vi "Resistance_SMUResistanceTest.vi"(7 "Published Data Id":T2, 9 "DCPower_Parameters":T1={"Output"=enum."DC Voltage", "Current_range"=0.0, "Current"=0.0, "Voltage_range"=0.0, "Voltage"=0.0, "Aperture_time"=0.0, "Source Delay"=0.0, "Sense"=1008} {"Source Delay" format="%.6p"; "Sense" items=["Local"=1008, "Remote"=1009]; "Aperture_time" format="%.6p"; "Current_range" format="%.6p"; "Current" format="%.6p"; "Voltage_range" format="%.6p"; "Voltage" format="%.6p"}, 10 "Pins":T3[](array[typedef]), 11 "Semiconductor Module Context":T4) -> (0 "error out":errorcluster)   [LabVIEW 2023, in "Resistance.lvlib"]
doc: "Measures the resistance using an SMU channel in order to perform simple Continuity Test"
uses:
  Resistance.lvlib
  <vilib>/NI_TestStand_SemiconductorModule/NI_TestStand_Semiconductor_Module.lvlibp/PinMap/General/SemiconductorModuleContext.ctl
  <vilib>/NI_TestStand_SemiconductorModule/NI_TestStand_Semiconductor_Module.lvlibp/PinMap/TagProvider/TSM_Pin.ctl
  <vilib>/NI_TestStand_SemiconductorModule/NI_TestStand_Semiconductor_Module.lvlibp/PinMap/TagProvider/TSM_PublishedDataId.ctl
  ResourceHandling/TypeDefs/RH_DCPower_Parameters.ctl
  <vilib>/NI_TestStand_SemiconductorModule/NI_TestStand_Semiconductor_Module.lvlibp/PinMap/DC Power/PinsToNIDCPowerSessions.vi
  <vilib>/NI_TestStand_SemiconductorModule/NI_TestStand_Semiconductor_Module.lvlibp/PinMap/General/Publish/PublishDataPerSiteDoubleScalar.vi
  ResourceHandling/ResourceHandling.lvlib
  <vilib>/NI_TestStand_SemiconductorModule/NI_TestStand_Semiconductor_Module.lvlibp
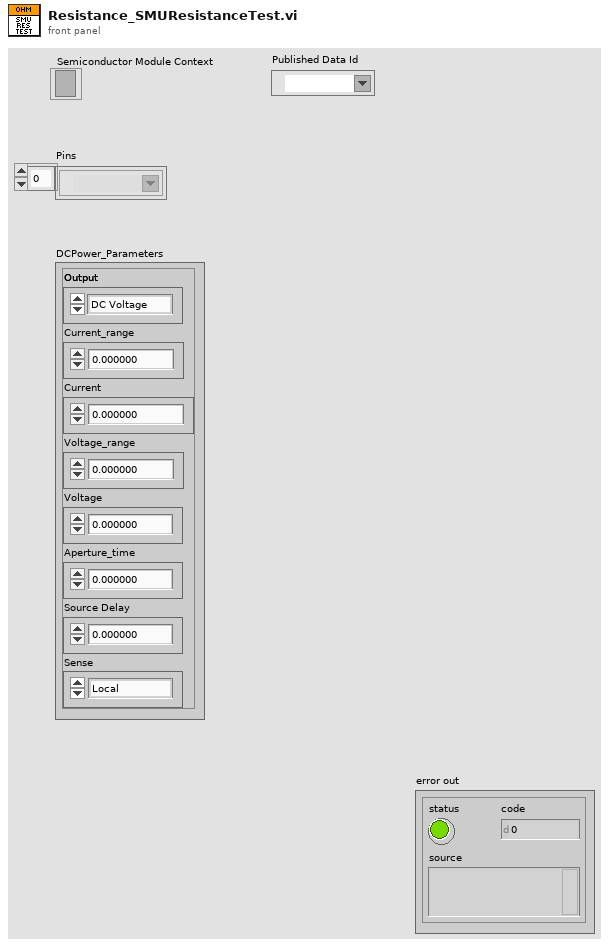
[diagram p1: front panel]
types:
  T1 = typedef "ResourceHandling.lvlib/RH_DCPower_Parameters.ctl" = cluster{"Output":enum16{"DC Voltage", "DC Current"}, "Current_range":dbl, "Current":dbl, "Voltage_range":dbl, "Voltage":dbl, "Aperture_time":dbl, "Source Delay":dbl, "Sense":i32}
  T2 = typedef "NI_TestStand_Semiconductor_Module.lvlibp/TSM_PublishedDataId.ctl" = tag
  T3 = typedef "NI_TestStand_Semiconductor_Module.lvlibp/TSM_Pin.ctl" = tag
  T4 = typedef "NI_TestStand_Semiconductor_Module.lvlibp/SemiconductorModuleContext.ctl" = refnum<k7>
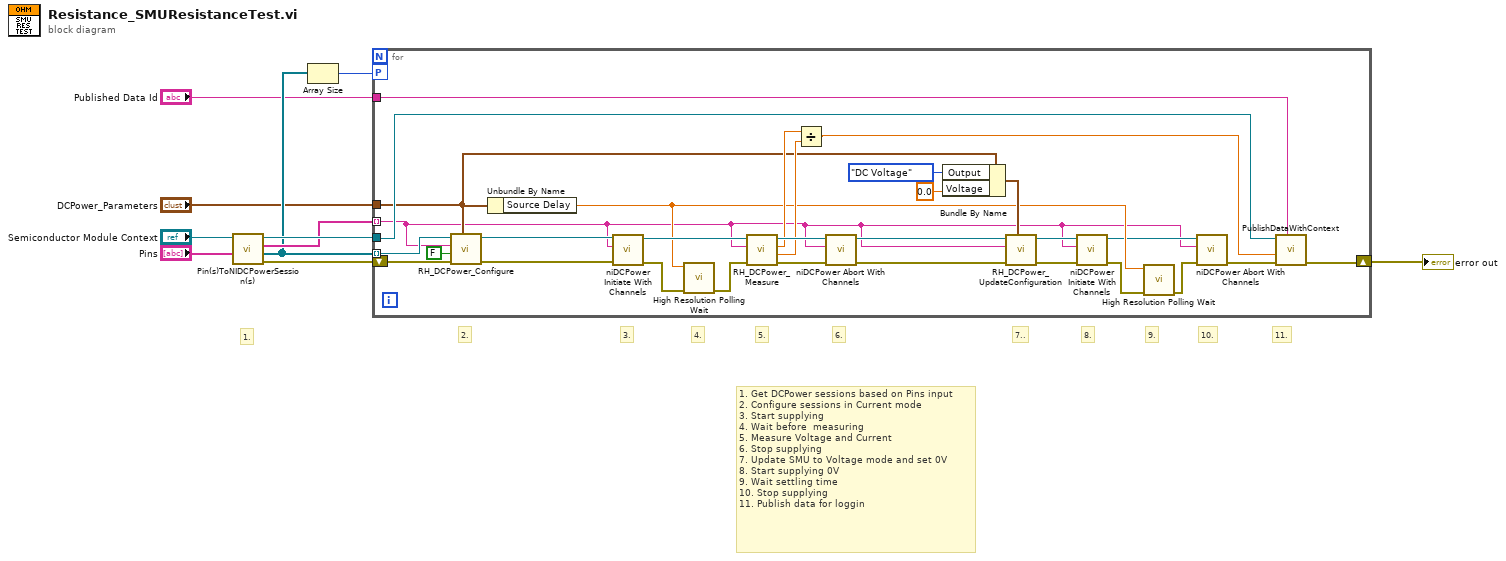
[diagram p0: block diagram]
diagram:
  # "11."
  # "10."
  # "9."
  # "8."
  # "1. Get DCPower sessions based on Pins input\n2. Configure sessions in Current mode\n3. Start supplying\n4. Wait before  measuring\n5. Measure Voltage and Current\n6. Stop supplying\n7. Update SMU to Voltage mode and set 0V\n8. Start supplying 0V\n9. Wait settling time\n10. Stop supplying\n11. Publish data for loggin"
  # "7.."
  # "6."
  # "5."
  # "4."
  # "3."
  # "2."
  # "1."
  n1 = call-poly <vilib>:"Pin(s)ToNIDCPowerSession(s).vi"("Pins"="Pins", "Semiconductor Module Context"="Semiconductor Module Context") -> ("error out"=w7:errorcluster, "Instrument Sessions"=w4:refnum<k15>[], "Channel Strings"=w6:string[], "Semiconductor Module Context Out"=w8:T4)  [unwired: 5 in, 1 out]
  n2 = Array Size(array=w4) -> (size(s)=w5:i32)
  n3 = for {
    tunnel: w8 -> [w32]
    shift-right: [w25] -> w3
    shift-left: w7 -> [w40]
    tunnel: w6 -> [w11] mode=indexing
    tunnel: w4 -> [w39] mode=indexing
    workers-P: w5 -> [_]
    tunnel: "DCPower_Parameters" -> [w22]
    tunnel: "Published Data Id" -> [w26]
    n4 = call "RH_DCPower_Configure.vi"("DCPower_Parameters"=w22, "error in (no error)"=w40, "trigger out?"=FALSE, "channel name"=w11, "DCPower Session In"=w39) -> ("error out"=w36:errorcluster, "DCPower Session Out"=w37:refnum<k15>)  [unwired: 5 in]
    n5 = Unbundle By Name(w22) -> ("Source Delay"=w15:dbl)
    n6 = call <instrlib>:"niDCPower Initiate With Channels.vi"("error in (no error)"=w36, "channel name"=w11, "instrument handle"=w37) -> ("error out"=w35:errorcluster, "instrument handle out"=w34:refnum<k15>)  [unwired: 7 in]
    n7 = call <vilib>:"High Resolution Polling Wait.vi"("error in (no error)"=w35, "seconds to wait"=w15) -> ("error out"=w33:errorcluster)  [unwired: 9 in]
    n8 = call "RH_DCPower_Measure.vi"("error in (no error)"=w33, "channel name"=w11, "DCPower Session In"=w34) -> ("error out"=w31:errorcluster, "Current"=w28:dbl, "Voltage"=w29:dbl, "DCPower Session Out"=w30:refnum<k15>)  [unwired: 5 in]
    n9 = Divide(x=w29, y=w28) -> (x/y=w27:dbl)
    n10 = call <instrlib>:"niDCPower Abort With Channels.vi"("error in (no error)"=w31, "channel name"=w11, "instrument handle"=w30) -> ("error out"=w24:errorcluster, "instrument handle out"=w23:refnum<k15>)  [unwired: 7 in]
    n11 = Bundle By Name(cluster=w22, "Output"=enum16{"DC Voltage", "DC Current"}."DC Voltage", "Voltage"=0.0) -> (w21:T1)
    n12 = call "RH_DCPower_UpdateConfiguration.vi"("DCPower_Parameters"=w21, "error in (no error)"=w24, "channel name"=w11, "DCPower Session In"=w23) -> ("error out"=w18:errorcluster, "DCPower Session Out"=w17:refnum<k15>)  [unwired: 6 in]
    n13 = call <instrlib>:"niDCPower Initiate With Channels.vi"("error in (no error)"=w18, "channel name"=w11, "instrument handle"=w17) -> ("error out"=w16:errorcluster, "instrument handle out"=w12:refnum<k15>)  [unwired: 7 in]
    n14 = call <vilib>:"High Resolution Polling Wait.vi"("error in (no error)"=w16, "seconds to wait"=w15) -> ("error out"=w14:errorcluster)  [unwired: 9 in]
    n15 = call <instrlib>:"niDCPower Abort With Channels.vi"("error in (no error)"=w14, "channel name"=w11, "instrument handle"=w12) -> ("error out"=w13:errorcluster)  [unwired: 7 in, 1 out]
    n16 = call-poly <vilib>:"PublishDataWithContext.vi"("Published Data Id"=w26, "error in (no error)"=w13, "Data In"=w27, "Semiconductor Module Context"=w32) -> ("error out"=w25:errorcluster)  [unwired: 6 in, 1 out]
  }
  "error out" <- w3
